vi "Do.vi"(8 "error in (no error)":errorcluster, 10 "Actor in":refnum<class "Actor.lvclass">, 11 "Receive Value Msg":refnum<class "Receive Value Msg.lvclass">) -> (0 "error out":errorcluster, 2 "Actor out":refnum<class "Actor.lvclass">)   [LabVIEW 2023, in "Abstraction.lvlib" / "Receive Value Msg.lvclass"]
doc: "This VI delivers the message to the actor by calling the appropriate method(s) on the actor."
uses:
  Receive Value Msg.lvclass
  <vilib>/ActorFramework/Actor/Actor.lvclass
  Abstraction/Abstraction.lvclass
  Receive Value Msg.lvclass/Receive Value Msg.ctl
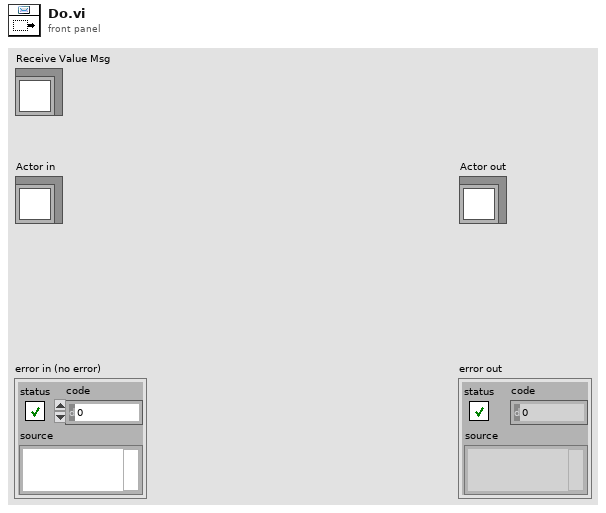
[diagram p1: front panel]
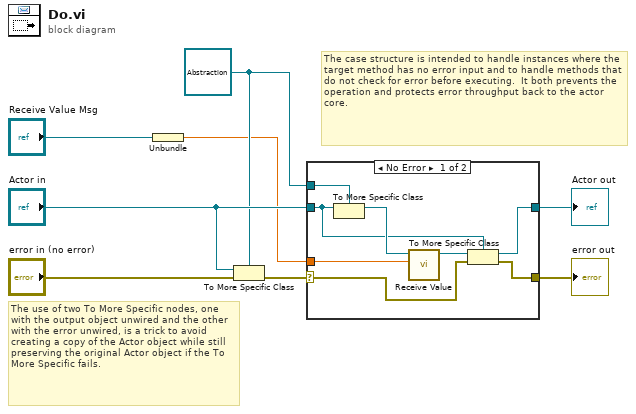
[diagram p0: block diagram]
diagram:
  w2 = refnum<class "Abstraction.lvclass"> refnum ("Actor in")
  # "The use of two To More Specific nodes, one with the output object unwired and the other with the error unwired, is a trick to avoid creating a copy of the Actor object while still preserving the original Actor object if the To More Specific fails."
  # "The case structure is intended to handle instances where the target method has no error input and to handle methods that do not check for error before executing.  It both prevents the operation and protects error throughput back to the actor core."
  n1 = Unbundle("Receive Value Msg") -> (w1:dbl)
  n2 = To More Specific Class(target class=w2, reference="Actor in", error in="error in (no error)") -> (error out=w6:errorcluster)  [unwired: 1 out]
  n3 = case shown="No Error" w6 {
    selector: w6 -> [w9 w18]
    tunnel: [w10 w18] -> w5
    tunnel: [w11 w17] -> w4
    tunnel: "Actor in" -> [w12 w17]
    tunnel: w2 -> [w16 _]
    tunnel: w1 -> [w14 _]
    frame No Error {
      n4 = To More Specific Class(target class=w16, reference=w12) -> (specific class reference=w15:refnum<class "Abstraction.lvclass">)  [unwired: 1 in, 1 out]
      n5 = call-dynamic "Receive Value.vi"("Numeric"=w14, "Abstraction in"=w15) -> ("Abstraction out"=w13:refnum<class "Abstraction.lvclass">)  [unwired: 9 in]
      n6 = To More Specific Class(target class=w12, reference=w13, error in=w9) -> (specific class reference=w11:refnum<class "Actor.lvclass">, error out=w10:errorcluster)
    }
    frame Error {
      # "If type check fails, pass the original object out again."
    }
  }
  "error out" <- w5
  "Actor out" <- w4
